vi "Choreo_SwerveSample_Interpolate.vi"(9 "TimeStamp":dbl, 10 "endValueSample":T1, 11 "ChoreoSwerveSample":T1) -> (3 "InterpolatedSample":T1)   [LabVIEW 2019, in "ChoreoLib.lvlib"]
doc: "Interpolate between two Swerve Trajectory Samples.\n\nInputs:\n -- ChoreoSwerveSample - cluster - Swerve sample.\n -- endChoreoSwerveSample - cluster - The end Swerve sample\n -- TimeStamp - double - desired time stamp\n\nOutputs:\n -- InterpolatedSample - cluster - Interpolated Swerve sample."
uses:
  ChoreoLib.lvlib
  TypeDef/ChoreoSwerveSample.ctl
  <vilib>/Rock Robotics/WPI/ThirdParty/JAS_Junk/TrajLib/MathUtil_Clamp.vi
  <vilib>/Rock Robotics/WPI/ThirdParty/JAS_Junk/TrajLib/Trajectory_Library.lvlib
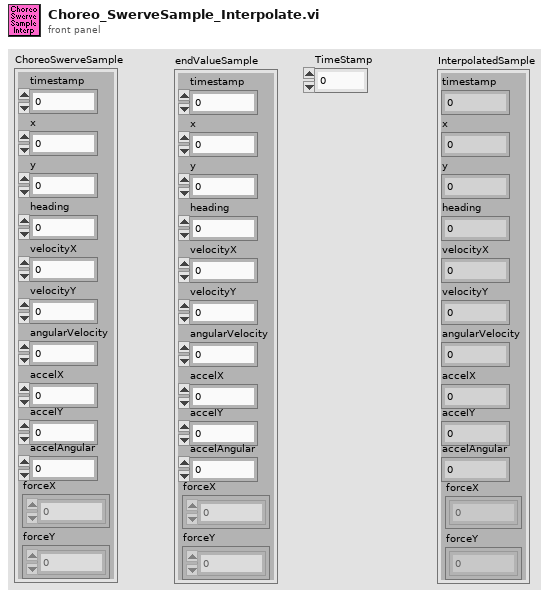
[diagram p1: front panel]
types:
  T1 = typedef "ChoreoLib.lvlib/ChoreoSwerveSample.ctl" = cluster{"timestamp":dbl, "x":dbl, "y":dbl, "heading":dbl, "velocityX":dbl, "velocityY":dbl, "angularVelocity":dbl, "accelX":dbl, "accelY":dbl, "accelAngular":dbl, "forceX":dbl[], "forceY":dbl[]}
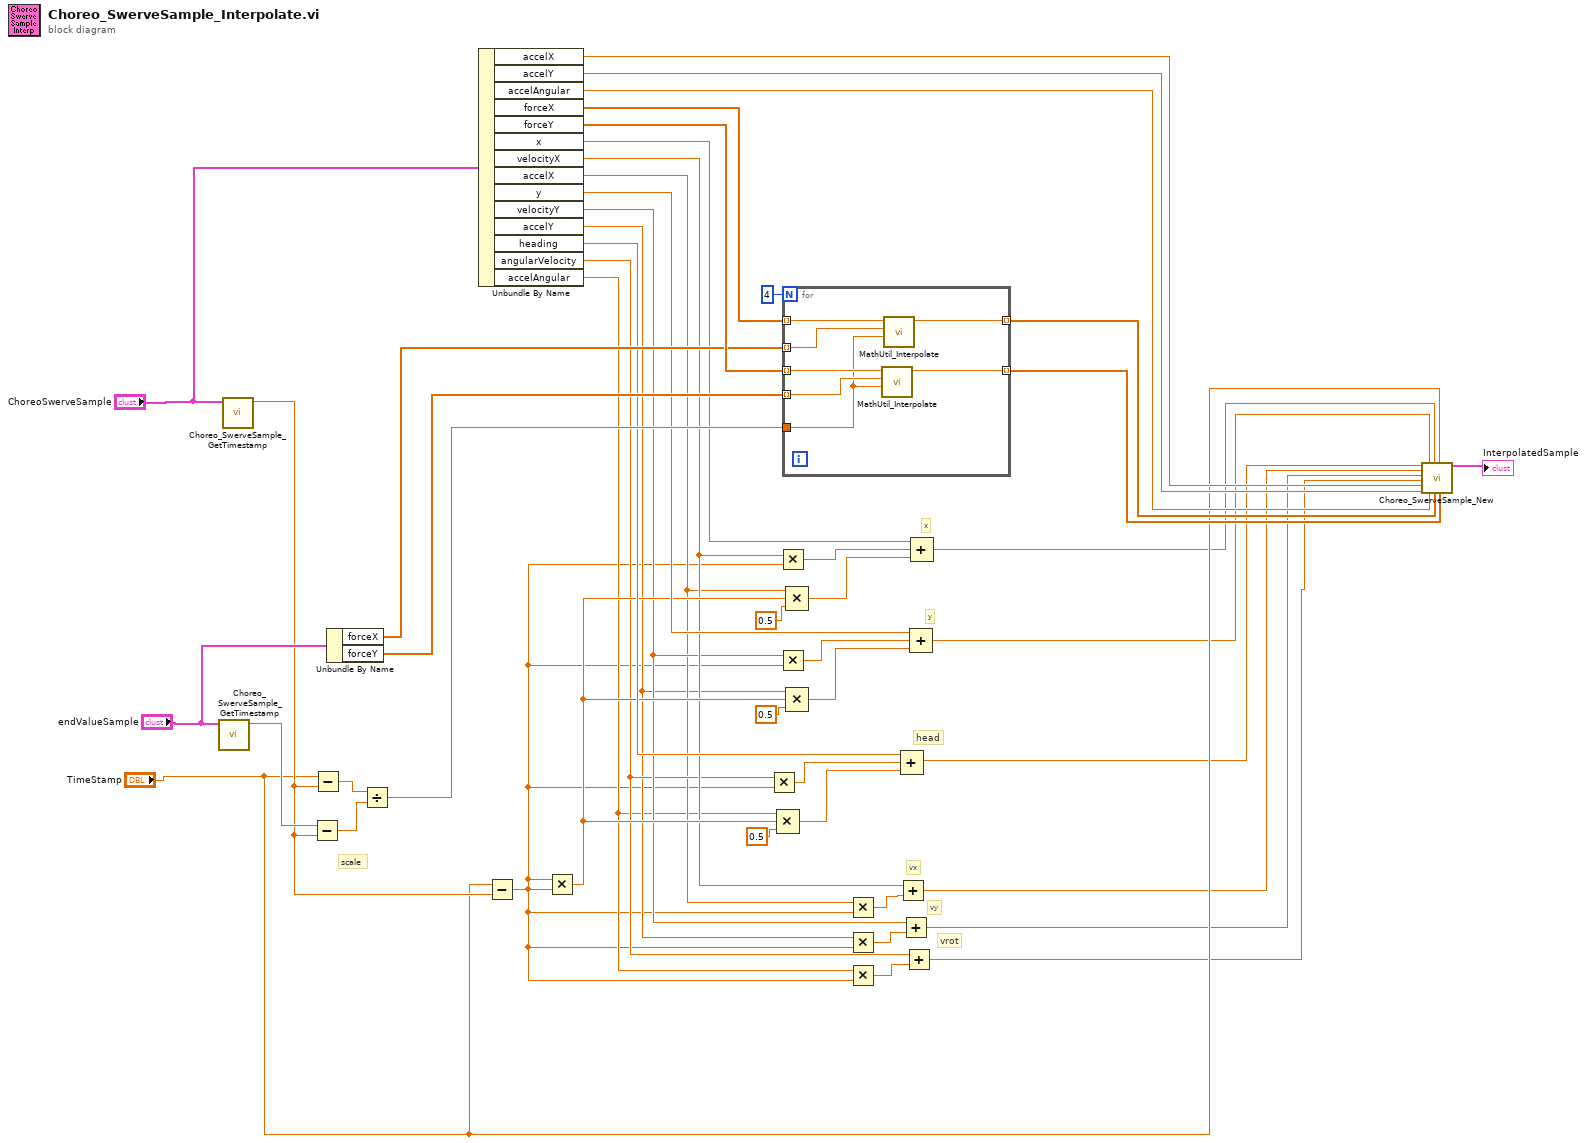
[diagram p0: block diagram]
diagram:
  # "vrot"
  # "vy"
  # "vx"
  # "head"
  # "y"
  # "x"
  # "scale"
  n1 = call "Choreo_SwerveSample_GetTimestamp.vi"("ChoreoSwerveSample"="endValueSample") -> ("Timestamp"=w48:dbl)  [unwired: 10 in]
  n2 = call "Choreo_SwerveSample_GetTimestamp.vi"("ChoreoSwerveSample"="ChoreoSwerveSample") -> ("Timestamp"=w35:dbl)  [unwired: 10 in]
  n3 = Subtract(x=w48, y=w35) -> (x-y=w46:dbl)
  n4 = Subtract(x="TimeStamp", y=w35) -> (x-y=w47:dbl)
  n5 = Unbundle By Name("endValueSample") -> ("forceX"=w39:dbl[], "forceY"=w30:dbl[])
  n6 = Divide(x=w47, y=w46) -> (x/y=w38:dbl)
  n7 = Unbundle By Name("ChoreoSwerveSample") -> ("accelX"=w32:dbl, "accelY"=w33:dbl, "accelAngular"=w34:dbl, "forceX"=w41:dbl[], "forceY"=w40:dbl[], "x"=w29:dbl, "velocityX"=w10:dbl, "accelX"=w7:dbl, "y"=w28:dbl, "velocityY"=w9:dbl, "accelY"=w6:dbl, "heading"=w17:dbl, "angularVelocity"=w8:dbl, "accelAngular"=w5:dbl)
  n8 = Subtract(x="TimeStamp", y=w35) -> (x-y=w4:dbl)
  n9 = Multiply(x=w4, y=w4) -> (x*y=w15:dbl)
  n10 = Multiply(x=w8, y=w4) -> (x*y=w16:dbl)
  n11 = Compound Arithmetic op=MULTIPLY(w5, w15, 0.5 ("value")) -> (w18:dbl)
  n12 = Multiply(x=w10, y=w4) -> (x*y=w25:dbl)
  n13 = Multiply(x=w9, y=w4) -> (x*y=w23:dbl)
  n14 = for {
    N: 4 -> [_]
    tunnel: w41 -> [w55] mode=indexing
    tunnel: w40 -> [w54] mode=indexing
    tunnel: w39 -> [w53] mode=indexing
    tunnel: w30 -> [w52] mode=indexing
    tunnel: w38 -> [w51]
    tunnel: [w50] -> w37 mode=indexing
    tunnel: [w49] -> w36 mode=indexing
    n15 = call <vilib>:"MathUtil_Interpolate.vi"("T"=w51, "EndValue"=w52, "StartValue"=w54) -> ("InterpolatedValue"=w50:dbl)  [unwired: 8 in]
    n16 = call <vilib>:"MathUtil_Interpolate.vi"("T"=w51, "EndValue"=w53, "StartValue"=w55) -> ("InterpolatedValue"=w49:dbl)  [unwired: 8 in]
  }
  n17 = Compound Arithmetic op=MULTIPLY(w7, w15, 0.5 ("value")) -> (w24:dbl)
  n18 = Compound Arithmetic op=MULTIPLY(w6, w15, 0.5 ("value")) -> (w22:dbl)
  n19 = Multiply(x=w7, y=w4) -> (x*y=w13:dbl)
  n20 = Multiply(x=w6, y=w4) -> (x*y=w12:dbl)
  n21 = Multiply(x=w5, y=w4) -> (x*y=w11:dbl)
  n22 = Add(x=w10, y=w13) -> (x+y=w3:dbl)
  n23 = Compound Arithmetic op=ADD(w17, w16, w18) -> (w14:dbl)
  n24 = Add(x=w9, y=w12) -> (x+y=w2:dbl)
  n25 = Add(x=w8, y=w11) -> (x+y=w1:dbl)
  n26 = Compound Arithmetic op=ADD(w28, w23, w22) -> (w20:dbl)
  n27 = Compound Arithmetic op=ADD(w29, w25, w24) -> (w21:dbl)
  n28 = call "Choreo_SwerveSample_New.vi"("heading"=w14, "velocityX"=w3, "velocityY"=w2, "angularVelocity"=w1, "accelX"=w32, "accelY"=w33, "y"=w20, "accelAngular"=w34, "x"=w21, "forceX"=w36, "timestamp"="TimeStamp", "forceY"=w37) -> ("ChoreoSwerveSample"=→"InterpolatedSample":T1)  [unwired: 7 in]
